vi "Toggle Intake and Grip.vi"(7 "Description":string, 8 "Command Info In":T1, 10 "Toggle intake":bool) -> (0 "Command Info Out":T1)   [LabVIEW 2019]
doc: "This template includes code for deadband comparision to avoid excessive command scheduling. It is particularly useful for joystick-driven commands.\n\nBe sure to right-click and select New from Template and save with a new command name."
uses:
  <vilib>/Rock Robotics/WPI/Framework/Command Status Info.ctl
  <vilib>/Rock Robotics/WPI/Framework/Completion Status.ctl
  <vilib>/Rock Robotics/WPI/Framework/Completion Notifier.ctl
  Implementation/Intake Setpoints.ctl
  Implementation/Intake Operations.ctl
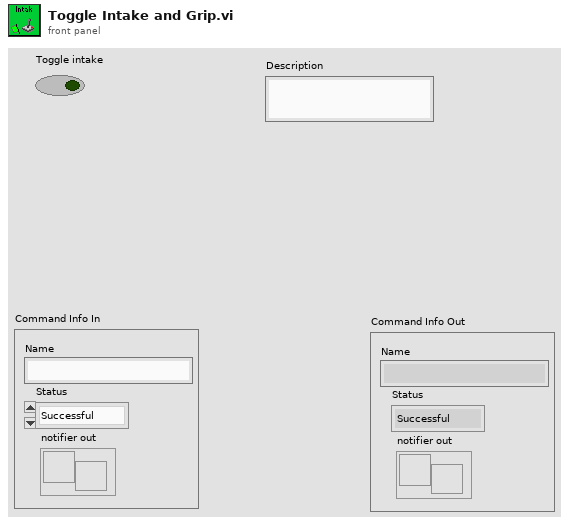
[diagram p1: front panel]
types:
  T1 = typedef "Command Status Info.ctl" = cluster{"Name":string, "Status":T2, "notifier out":T3}
  T2 = typedef "Completion Status.ctl" = enum16{"Successful", "Aborted", "Incomplete"}
  T3 = typedef "Completion Notifier.ctl" = refnum<notifier>
  T4 = typedef "Intake Setpoints.ctl" = cluster{"Operation":T5, "Toggle intake":bool}
  T5 = typedef "Intake Operations.ctl" = enum16{"Reserve", "Read Current", "Immediate", "Toggle Intake", "Gripper"}
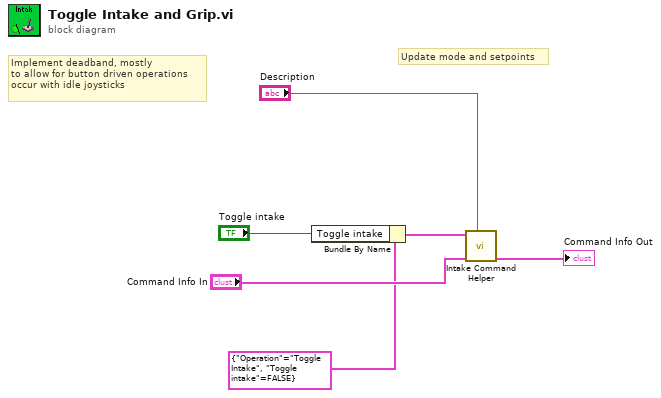
[diagram p0: block diagram]
diagram:
  # "Implement deadband, mostly\nto allow for button driven operations\noccur with idle joysticks"
  # "Update mode and setpoints"
  n1 = Bundle By Name(cluster=T4 {"Operation"=enum."Toggle Intake", "Toggle intake"=FALSE} ("SubSystem Data"), "Toggle intake"="Toggle intake") -> (w3:T4)
  n2 = call "Intake Command Helper.vi"("Description"="Description", "Command Info In"="Command Info In", "SubSystem Data"=w3) -> ("Command Info Out"=→"Command Info Out":T1)  [unwired: 6 in, 2 out]
